vi "Get ECAT Reconfig Status.vi"(8 "error in (no error)":errorcluster, 10 "timeout in ms (0)":i32, 11 "Status in":refnum<queue>) -> (0 "error out":errorcluster, 2 "State":T1, 3 "Status out":refnum<queue>)   [LabVIEW 2019, in "SEECD Engine.lvlib"]
uses:
  SEECD Engine.lvlib
  Type Defs/ECAT Reconfig State.ctl
  Type Defs/ECAT Reconfig Status.ctl
  Shared/Globals/Error Strings.vi
  Shared/SEECD Shared.lvlib
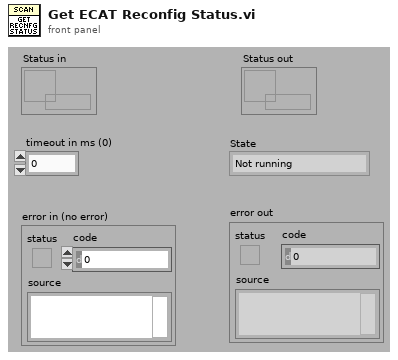
[diagram p1: front panel]
types:
  T1 = typedef "SEECD Engine.lvlib/ECAT Reconfig State.ctl" = enum16{"Not running", "Waiting to Start", "Started", "Running"}
  T2 = typedef "SEECD Engine.lvlib/ECAT Reconfig Status.ctl" = cluster{"State":T1, "error":errorcluster}
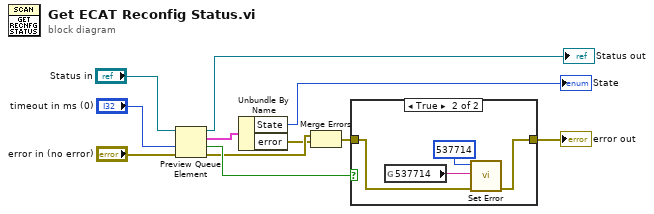
[diagram p0: block diagram]
diagram:
  n1 = Preview Queue Element(queue="Status in", timeout in ms (-1)="timeout in ms (0)", error in (no error)="error in (no error)") -> (queue out=→"Status out":refnum<queue>, element=w11:T2, timed out?=w8:bool, error out=w3:errorcluster)
  n2 = Unbundle By Name(w11) -> ("State"=→"State":T1, "error"=w2:errorcluster)
  n3 = Merge Errors(w3, w2) -> (w1:errorcluster)
  n4 = case shown="True" w8 {
    tunnel: [w12 w15] -> w7
    tunnel: w1 -> [w12 w16]
    frame False {
    }
    frame True {
      n5 = global read "Error Strings.vi" "537714"() -> (w13:string)
      n6 = call "Set Error.vi"("error in (no error)"=w16, "Message"=w13, "Code"=537714 ("code")) -> ("error out"=w15:errorcluster)  [unwired: 8 in]
    }
  }
  "error out" <- w7
